vi "Get Wfm Path from WfmStreamSpec.vi"(8 "error in (no error)":errorcluster, 11 ".NET Refnum in":T1) -> (0 "error out":errorcluster, 2 "WaveformPath":string, 3 ".NET Refnum out":T1, 5 "WaveformPath (Duplicate)":string)   [LabVIEW 2020, in "FPGA Addon DMA Channels Basic System Tests.lvclass"]
uses:
  FPGA Addon DMA Channels Basic System Tests.lvclass
  FPGA Addon DMA Channels Basic System Tests.lvclass/FPGA Addon DMA Channels Basic System Tests.ctl
  NationalInstruments.VeriStand.ClientAPI
  <vilib>/NI VeriStand/Execution/WaveformStreaming/WaveformStreamSpecification.ctl
  <vilib>/NI VeriStand/Execution/WaveformStreaming/NI_VS Waveform Streaming Interface.lvlib
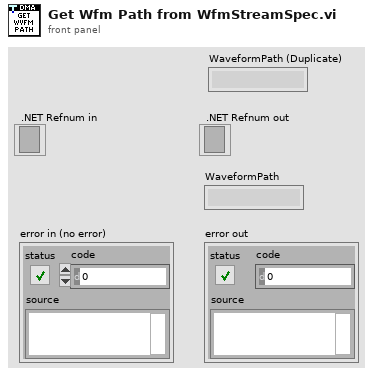
[diagram p1: front panel]
types:
  T1 = typedef "NI_VS Waveform Streaming Interface.lvlib/WaveformStreamSpecification.ctl" = refnum<k24>
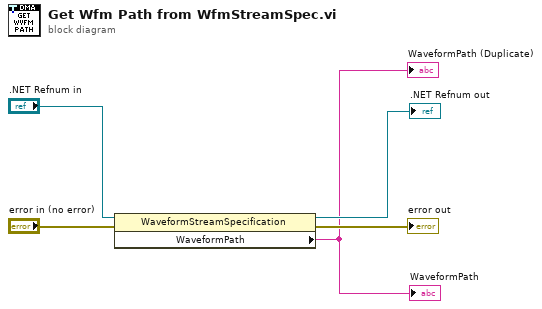
[diagram p0: block diagram]
diagram:
  n1 = property class="WaveformStreamSpecification"(reference=".NET Refnum in", error in="error in (no error)") -> (reference out=→".NET Refnum out":T1, error out=→"error out":errorcluster, "WaveformPath"=→"WaveformPath" →"WaveformPath (Duplicate)":string)
